vi "ConvertMessageStringToBytes.vi"(11 "8x8MessageString":string) -> (3 "BytesOut":u8[](array[numeric]) format="%.0x")   [LabVIEW 2020, in "CTI-Peripheral.lvlib"]
uses:
  CTI-Peripheral.lvlib
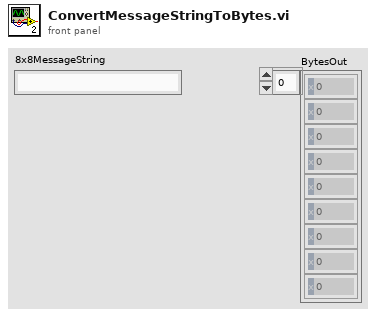
[diagram p1: front panel]
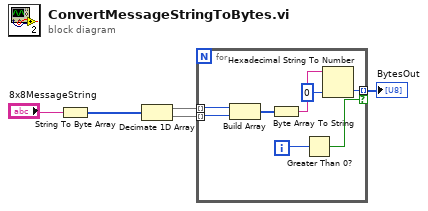
[diagram p0: block diagram]
diagram:
  n1 = String To Byte Array(string="8x8MessageString") -> (unsigned byte array=w4:u8[])
  n2 = Decimate 1D Array(w4) -> (w3:u8[], w2:u8[])
  n3 = for {
    tunnel: w3 -> [w13] mode=indexing
    tunnel: w2 -> [w12] mode=indexing
    tunnel: [w7] -> w1 mode=indexing if=w6
    i -> [w10]
    n4 = Build Array(w13, w12) -> (w11:u8[])
    n5 = Byte Array To String(unsigned byte array=w11) -> (string=w9:string)
    n6 = Greater Than 0?(x=w10) -> (x > 0?=w6:bool)
    n7 = Hexadecimal String To Number(string=w9, default (0uL)=u8 0 ("default (0 U32)")) -> (number=w7:u8)  [unwired: 1 in, 1 out]
  }
  "BytesOut" <- w1
